vi "MotionMacro@WaitMotor(Combine)__Parameter.vi"(1 "ParamterIn":string) -> (0 "ParamterOut":string)   [LabVIEW 2020]
panel:
  in  "Message":string(combo)
  in  "TimeOut":string(combo)
  in  "MotorSelect":string(combo)
  in  "Confirm":bool
  # "Motion@WaitMotor $Motor(,$Timeout=XX,[[$label]]$Message)"
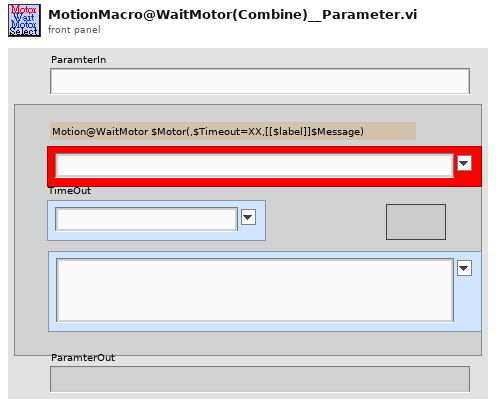
[diagram p1: front panel]
types:
  T1 = enum16{"Get", "Init", "Set", "Delete", "GetElement", "Inc", "Dec", "ReName", "Copy"}
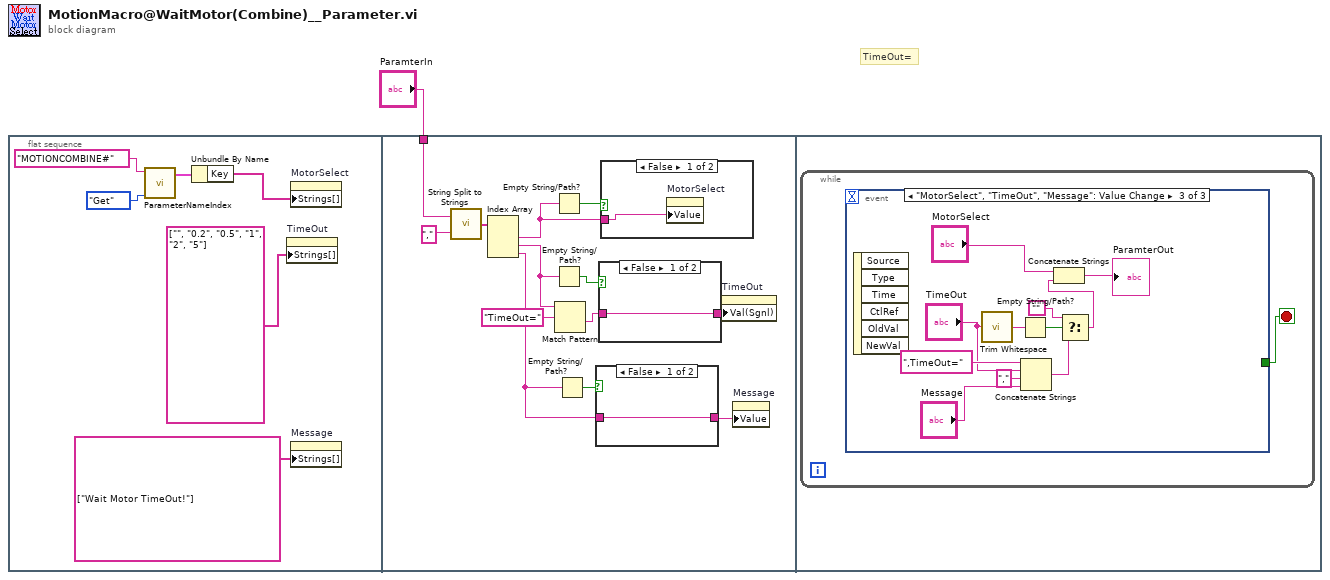
[diagram p0: block diagram]
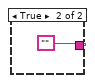
[diagram p2: hidden frame]
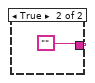
[diagram p3: hidden frame]
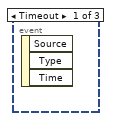
[diagram p5: hidden frame]
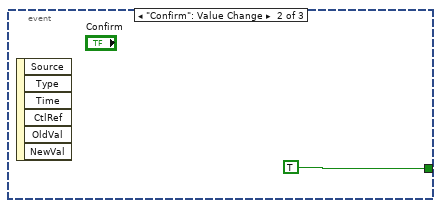
[diagram p6: hidden frame]
diagram:
  # "TimeOut="
  n1 = flat-sequence {
    tunnel: "ParamterIn" -> [w18]
    frame #0 {
      n2 = call "ParameterNameIndex.vi"("OP"=T1."Get", "VariableSection"="MOTIONCOMBINE#" ("string")) -> ("SectionKeyValue"=w4:cluster{"Key":string[], "Value":string[]})  [unwired: 3 in, 6 out]
      n3 = Unbundle By Name(w4) -> ("Key"=w2:string[])
      n4 = property on="TimeOut" class="CmbBox"("Strings[]"=string[] ["", "0.2", "0.5", "1", "2", "5"] ("Strings []")) -> ()  [unwired: 2 in, 2 out]
      n5 = property on="MotorSelect" class="CmbBox"("Strings[]"=w2) -> ()  [unwired: 2 in, 2 out]
      n6 = property on="Message" class="CmbBox"("Strings[]"=string[] ["Wait Motor TimeOut!"] ("Strings []")) -> ()  [unwired: 2 in, 2 out]
    }
    frame #1 {
      n7 = call "String Split to Strings.vi"("search string/char (-)"=",", "String"=w18) -> ("Array"=w20:string[])
      n8 = Index Array(array=w20) -> (element #1=w16:string, element #2=w13:string, element #3=w9:string)  [unwired: 3 in]
      n9 = Empty String/Path?(string/path=w16) -> (empty?=w17:bool)
      n10 = Empty String/Path?(string/path=w13) -> (empty?=w15:bool)
      n11 = Match Pattern(string=w13, regular expression="TimeOut=") -> (after substring=w11:string)  [unwired: 1 in, 3 out]
      n12 = Empty String/Path?(string/path=w9) -> (empty?=w10:bool)
      n13 = case shown="False" w10 {
        tunnel: [w21 ""] -> w8
        tunnel: w9 -> [w21 _]
        frame False {
        }
        frame True {
        }
      }
      n14 = case shown="False" w15 {
        tunnel: [w23 ""] -> w14
        tunnel: w11 -> [w23 _]
        frame False {
        }
        frame True {
        }
      }
      n15 = case shown="False" w17 {
        tunnel: w16 -> [w25 _]
        frame False {
          n16 = property on="MotorSelect" class="CmbBox"("Value"=w25) -> ()  [unwired: 2 in, 2 out]
        }
        frame True {
        }
      }
      n17 = property on="TimeOut" class="CmbBox"("Val(Sgnl)"=w14) -> ()  [unwired: 2 in, 2 out]
      n18 = property on="Message" class="CmbBox"("Value"=w8) -> ()  [unwired: 2 in, 2 out]
    }
    frame #2 {
      n19 = while {
        stop <- w26 stop-if-true
        n20 = event shown="[2] \"MotorSelect\", \"TimeOut\", \"Message\": Value Change" {
          selector: _ -> [_ _ _]
          dyn-events: _ -> [_ _ _]
          timeout: _ -> [_ _ _]
          tunnel: [_ TRUE _] -> w26
          event Timeout {
            n21 = event-data() -> ()  [unwired: 1 in, 3 out]
          }
          event "Confirm": Value Change {
            n22 = event-data() -> ()  [unwired: 1 in, 6 out]
          }
          event "MotorSelect", "TimeOut", "Message": Value Change {
            n23 = event-data() -> ()  [unwired: 1 in, 6 out]
            n24 = call <vilib>:"Trim Whitespace.vi"("string"="TimeOut") -> ("trimmed string"=w32:string)  [unwired: 1 in]
            n25 = Empty String/Path?(string/path=w32) -> (empty?=w33:bool)
            n26 = Concatenate Strings(",TimeOut=" ("string"), "TimeOut", "," ("string"), "Message") -> (w35:string)
            n27 = Select(t="", s=w33, f=w35) -> (s? t:f=w30:string)
            n28 = Concatenate Strings("MotorSelect", w30) -> (→"ParamterOut":string)
          }
        }
      }
    }
  }
